vi "Auto Mode.vi"(11 "Ball?":bool) -> ()   [LabVIEW 2016]
uses:
  <vilib>/Rock Robotics/WPI/Camera/WPI_CameraExposure Values.ctl
  <vilib>/Rock Robotics/WPI/Camera/WPI_CameraWhite Balance Values.ctl
  <vilib>/Rock Robotics/Network Tables/NT Write Boolean.vi
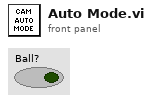
[diagram p1: front panel]
types:
  T1 = typedef "WPI_CameraDevRef.ctl" = cluster{"Camera Address":string, "CameraStatus":errorcluster}
  T2 = typedef "WPI_CameraWhite Balance Values.ctl" = enum16{"Auto", "Fixed indoor", "Fixed outdoor 1", "Fixed outdoor 2", "Fixed fluorescent 1", "Fixed fluorescent 2", "Hold current", "Custom"}
  T3 = typedef "WPI_CameraExposure Values.ctl" = enum16{"Auto", "Flicker-free 50 Hz", "Flicker-free 60 Hz", "Hold current", "Custom"}
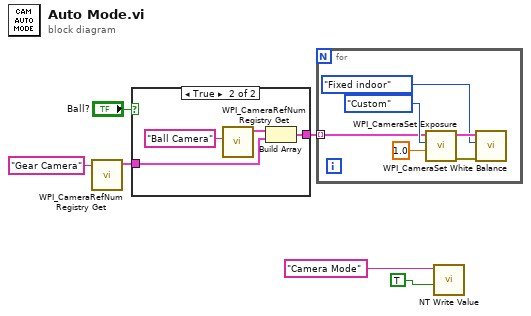
[diagram p0: block diagram]
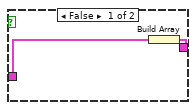
[diagram p2: hidden frame]
diagram:
  n1 = call <vilib>:"WPI_CameraRefNum Registry Get.vi"("refnum name"="Gear Camera") -> ("CameraDevRef"=w1:T1)  [unwired: 9 in, 1 out]
  n2 = case shown="True" "Ball?" {
    tunnel: w1 -> [w8 w11]
    tunnel: [w7 w10] -> w2
    frame False {
      n3 = Build Array(w8) -> (w7:T1[])
    }
    frame True {
      n4 = call <vilib>:"WPI_CameraRefNum Registry Get.vi"("refnum name"="Ball Camera") -> ("CameraDevRef"=w9:T1)  [unwired: 9 in, 1 out]
      n5 = Build Array(w9, w11) -> (w10:T1[])
    }
  }
  n6 = for {
    tunnel: w2 -> [w16] mode=indexing
    n7 = call <vilib>:"WPI_CameraSet Exposure.vi"("Exposure (%)"=1.0, "Exposure"=WPI_CameraExposure_Values."Custom", "CameraDevRef"=w16) -> ("error out"=w13:errorcluster, "CameraDevRef Out"=w15:T1)  [unwired: 1 in, 6 out]
    n8 = call <vilib>:"WPI_CameraSet White Balance.vi"("error in (no error)"=w13, "White Balance"=WPI_CameraWhite_Balance_Values."Fixed indoor", "CameraDevRef"=w15) -> ()  [unwired: 1 in, 8 out]
  }
  n9 = call-poly <vilib>:"NT Write Value.vi"("Boolean"=TRUE, "Name"="Camera Mode") -> ()  [unwired: 9 in, 1 out]
